vi "Write Data.vi"(10 "Data":i32, 11 "Main UI Task Msg in":refnum<class "Main UI Task Msg.lvclass">) -> (3 "Main UI Task Msg out":refnum<class "Main UI Task Msg.lvclass">)   [LabVIEW 2016, in "Main UI Actor.lvlib" / "Main UI Task Msg.lvclass"]
uses:
  Main UI Task Msg.lvclass
  Main UI Task Msg.lvclass/Main UI Task Msg.ctl
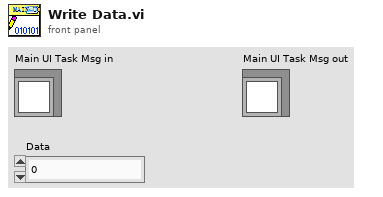
[diagram p1: front panel]
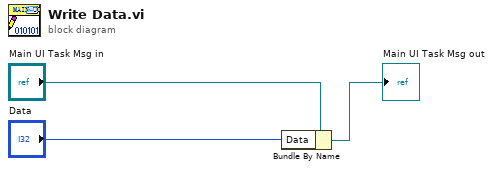
[diagram p0: block diagram]
diagram:
  n1 = Bundle By Name(cluster="Main UI Task Msg in", "Data"="Data") -> (→"Main UI Task Msg out":refnum<class "Main UI Task Msg.lvclass">)
